vi "test Get Array Size - Empty Array.vi"(8 "error in (no error)":errorcluster, 11 "TestCase in":refnum<class "Python String Parsing Utility Tests.lvclass">) -> (0 "error out":errorcluster, 3 "TestCase out":refnum<class "Python String Parsing Utility Tests.lvclass">)   [LabVIEW 2020, in "Python String Parsing Utility Tests.lvclass"]
uses:
  Python String Parsing Utility Tests.lvclass
  Python String Parsing Utility Tests.lvclass/Python String Parsing Utility Tests.ctl
  <vilib>/addons/_JKI Toolkits/VI Tester/TestCase.llb/TestCase.lvclass
  source/jki_python_data_tools.lvlib
  C:/Program Files/National Instruments/LabVIEW 2020/vi.lib/addons/_JKI Toolkits/VI Tester/TestCase.llb/TestCase.lvclass
panel:
  out "Python String out":string
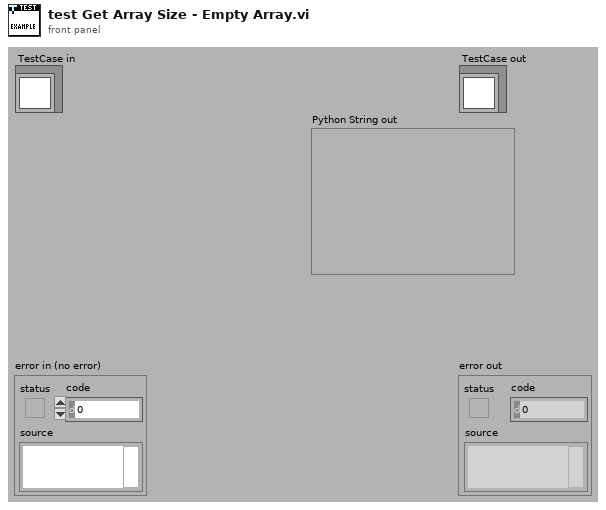
[diagram p1: front panel]
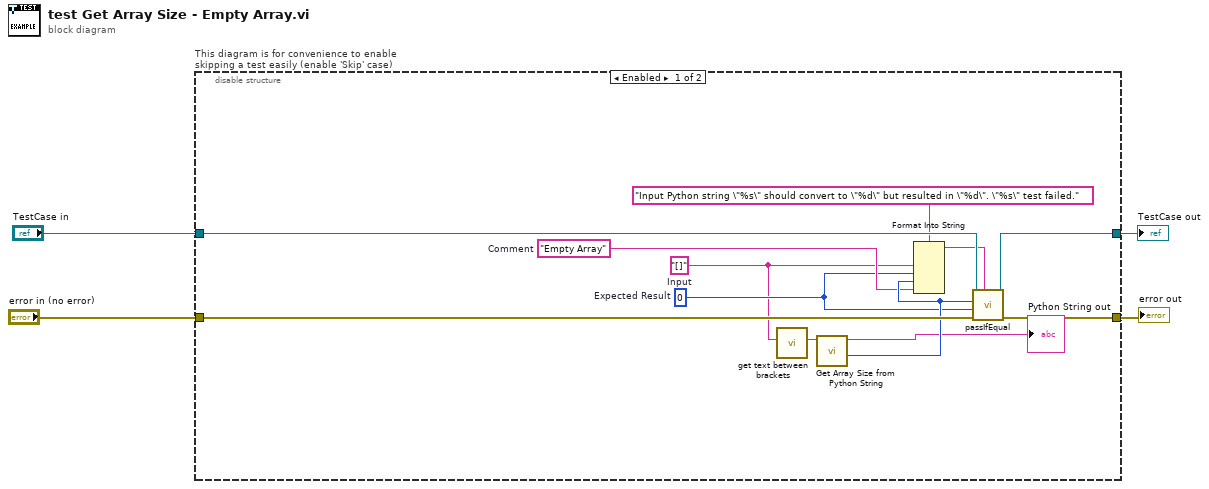
[diagram p0: block diagram]
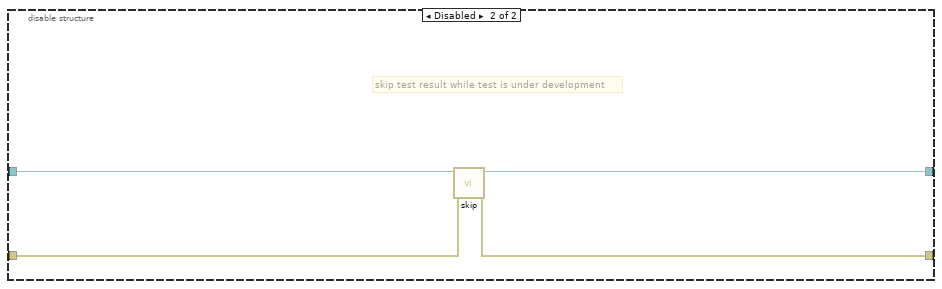
[diagram p2: hidden frame]
diagram:
  n1 = disable-structure "This diagram is for convenience to enable skipping a test easily (enable 'Skip' case)" shown="Enabled" {
    disable-tunnel: "TestCase in" -> [w16 w20]
    disable-tunnel: [w14 w18] -> w1
    disable-tunnel: [w13 w19] -> w3
    disable-tunnel: "error in (no error)" -> [w15 w17]
    frame Enabled {
      w9 = "Empty Array"  # Comment
      w8 = 0  # Expected Result
      w7 = "[]"  # Input
      n2 = call "get text between brackets.vi"("Python String"=w7) -> ("Text Between Brakets"=w6:string)  [unwired: 10 in]
      n3 = call "Get Array Size from Python String.vi"("Python String"=w6) -> ("Array Size"=w10:i32, "Python String out"=→"Python String out":string)  [unwired: 9 in]
      n4 = Format Into String(format string="Input Python string \"%s\" should convert to \"%d\" but resulted in \"%d\". \"%s\" test failed.", w7, w8, w10, w9) -> (resulting string=w12:string)  [unwired: 2 in, 1 out]
      n5 = call-dynamic "passIfEqual.vi"("custom report message (\"\")"=w12, "error in (no error)"=w15, "y"=w8, "x"=w10, "TestCase in"=w16) -> ("error out"=w13:errorcluster, "TestCase out"=w14:refnum<class "Python String Parsing Utility Tests.lvclass">)  [unwired: 5 in]
    }
    frame Disabled {
      # "skip test result while test is under development"
      n6 = call <vilib>:"skip.vi"("error in (no error)"=w17, "TestCase in"=w20) -> ("error out"=w19:errorcluster, "TestCase out"=w18:refnum<class "Python String Parsing Utility Tests.lvclass">)  [unwired: 8 in]
    }
  }
  "error out" <- w3
  "TestCase out" <- w1
